vi "Send Abort [TRG].vi"(7 "Message Priority (Normal)":T1=enum."Normal", 8 "error in (no error)":errorcluster, 11 "Message Enqueuer":refnum<class "Message Enqueuer.lvclass">) -> (0 "error out":errorcluster, 3 "Message Enqueuer out":refnum<class "Message Enqueuer.lvclass">)   [LabVIEW 2015, in "CS++DCPwr.lvlib" / "Abort [TRG] Msg.lvclass"]
doc: "Sends the <B>CS++DCPwr.lvlib:Abort [TRG] Msg.lvclass</B> message.\n\n<B>CS++DCPwr.lvlib:CS++DCPwr.lvclass:Abort [TRG].vi</B> Description:\n\nThis VI aborts all pending output changes.\n\nNotes:\n\n(1) This VI is part of the IviDCPwrTrigger [TRG] extension group.\n\n(2) If you call this VI after calling the IviDCPwr Initiate [TRG] VI, the power supply ignores any trigger and does not change the output."
uses:
  Abort [TRG] Msg.lvclass
  <vilib>/ActorFramework/Message Enqueuer/Message Enqueuer.lvclass
  <vilib>/ActorFramework/Message Enqueuer/Message Priority.ctl
  <vilib>/ActorFramework/Message Enqueuer/Message Enqueuer.lvclass/Message Enqueuer.ctl
  <vilib>/ActorFramework/Message Priority Queue/Priority Enqueue.vi
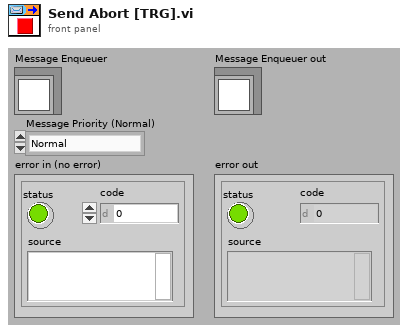
[diagram p1: front panel]
types:
  T1 = typedef "Actor Framework.lvlib/Message Enqueuer.lvclass/Message Priority.ctl" = enum16{"Low", "Normal", "High"}
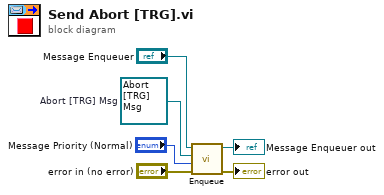
[diagram p0: block diagram]
diagram:
  w1 = refnum<class "Abort [TRG] Msg.lvclass"> refnum  # Abort [TRG] Msg
  n1 = call <vilib>:"Enqueue.vi"("error in (no error)"="error in (no error)", "Message Priority (Normal)"="Message Priority (Normal)", "Message"=w1, "Message Enqueuer in"="Message Enqueuer") -> ("error out"=→"error out":errorcluster, "Message Enqueuer out"=→"Message Enqueuer out":refnum<class "Message Enqueuer.lvclass">)  [unwired: 6 in]
